vi "GetPlugin.vi"() -> (3 "Plugin":refnum<class "Base.lvclass">)   [LabVIEW 2014, in "Plugin1.lvlib"]
uses:
  Plugin1.lvlib
  Framework/Base.lvclass
  Plugin1.lvclass
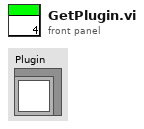
[diagram p1: front panel]
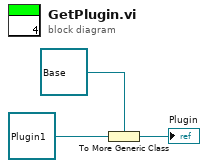
[diagram p0: block diagram]
diagram:
  n1 = To More Generic Class(target class=refnum<class "Base.lvclass"> refnum ("Framework.lvlib:Base.lvclass"), reference=refnum<class "Plugin1.lvclass"> refnum ("Plugin1.lvlib:Plugin1")) -> (generic class reference=→"Plugin":refnum<class "Base.lvclass">)
